vi "User_Defined_Test_InverseKinematics.vi"() -> (3 "Unit Test Framework Results":T1)   [LabVIEW 2016]
doc: "Use this template to create a user-defined test VI. Define your test requirements and wire the results to the <b>Result (Test)</b> control. Do not modify the <b>Unit Test Framework Results</b> indicator."
uses:
  <vilib>/utf/common/utf_test_result_troll.ctl
  <vilib>/utf/common/utf_test_result.ctl
  <vilib>/utf/common/utf_test_result_failure.ctl
  <vilib>/utf/common/utf_test_comparison_operators.ctl
  <vilib>/utf/common/utf_vi_tag.ctl
  <vilib>/Control Software Solutions Ltd/UTF Helper/SubVIs/UTF Double Equals.vi
  MyPAM Controller/controllerLibrary.lvlib
  <vilib>/Control Software Solutions Ltd/UTF Helper/Unit Test Helper.lvlib
  <vilib>/utf/NI_UnitTestFramework.lvlib
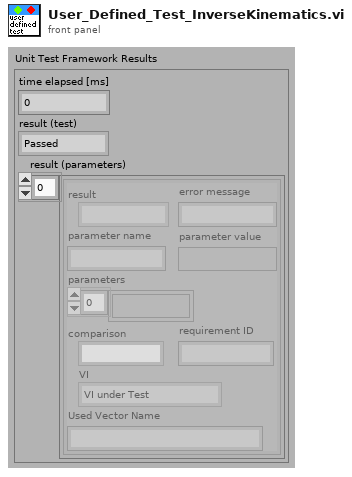
[diagram p1: front panel]
types:
  T1 = typedef "NI_UnitTestFramework.lvlib/utf_test_result_troll.ctl" = cluster{"time elapsed [ms]":u32, "result (test)":T2, "result (parameters)":T3[]}
  T2 = typedef "NI_UnitTestFramework.lvlib/utf_test_result.ctl" = enum16{"Passed", "Failed", "Error", "Skipped", "Not Processed"}
  T3 = typedef "NI_UnitTestFramework.lvlib/utf_test_result_failure.ctl" = cluster{"result":T2, "error message":string, "parameter name":string, "parameter value":variant, "parameters":variant[], "comparison":T4, "requirement ID":string, "VI":T5, "Used Vector Name":string}
  T4 = typedef "NI_UnitTestFramework.lvlib/utf_test_comparison_operators.ctl" = enum16{"=", "!=", ">", ">=", "<", "<=", "range", "symmetric tolerance", "asymmetric tolerance", "string contains", "string not contain", "array size", "string length", "array range", "by element", "array range (limit array)", "user-defined", "array contains", "array not contain", "vector length", "= (elm)", "!= (elm)", "= (case insensitive)", "!= (case insensitive)"}
  T5 = typedef "NI_UnitTestFramework.lvlib/utf_vi_tag.ctl" = enum16{"Setup VI", "VI under Test", "Teardown VI"}
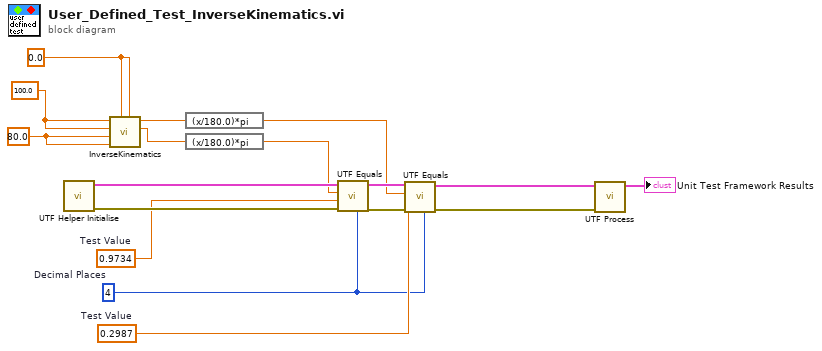
[diagram p0: block diagram]
diagram:
  w8 = 0.2987  # Test Value
  w7 = u8 4  # Decimal Places
  w11 = 0.9734  # Test Value
  w14 = 0.0 ("deltaY")
  w15 = 80.0 ("L0")
  w16 = 100.0 ("Next X")
  n1 = call <vilib>:"UTF Helper Initialise.vi"() -> ("error out"=w12:errorcluster, "results array"=w13:T3[])  [unwired: 10 in]
  n2 = call "InverseKinematics.vi"("deltaX"=w14, "deltaY"=w14, "L1"=w15, "L0"=w15, "Next Y"=w16, "Next X"=w16) -> ("theta1"=w2:dbl, "theta0"=w4:dbl)  [unwired: 4 in]
  n3 = expression code="(x/180.0)*pi" ("degrees to radians")(w4) -> (w3:dbl)
  n4 = expression code="(x/180.0)*pi" ("degrees to radians")(w2) -> (w1:dbl)
  n5 = call-poly <vilib>:"UTF Equals.vi"("Decimal Places"=w7, "error in (no error)"=w12, "Test Value"=w11, "Input"=w1, "Input Results"=w13) -> ("error out"=w9:errorcluster, "Output Results"=w10:T3[])  [unwired: 5 in]
  n6 = call-poly <vilib>:"UTF Equals.vi"("Decimal Places"=w7, "error in (no error)"=w9, "Test Value"=w8, "Input"=w3, "Input Results"=w10) -> ("error out"=w5:errorcluster, "Output Results"=w6:T3[])  [unwired: 5 in]
  n7 = call <vilib>:"UTF Process.vi"("error in (no error)"=w5, "results array"=w6) -> ("Unit Test Framework Results"=→"Unit Test Framework Results":T1)  [unwired: 9 in]
